vi "Edge Counting DAQ Assistant.vi"() -> ()   [LabVIEW 2020]
panel:
  out "Scalar":dbl
  in  "stop (F)":bool
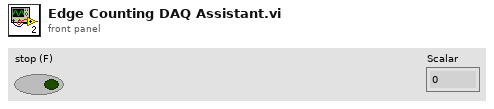
[diagram p1: front panel]
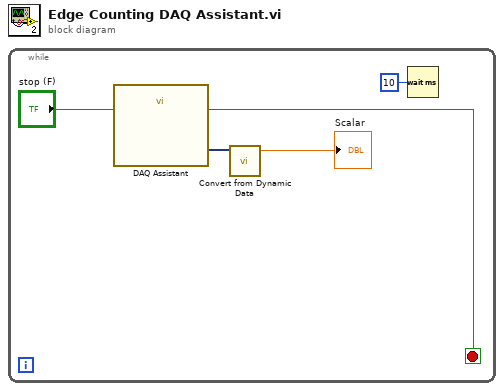
[diagram p0: block diagram]
diagram:
  n1 = while {
    stop <- w4 stop-if-true
    n2 = call "DAQ Assistant"("stop (F)"="stop (F)") -> ("data"=w3:dynamicdata, "stopped"=w4:bool)  [unwired: 15 in, 2 out]
    n3 = call "Convert from Dynamic Data"("Dynamic Data Type"=w3) -> ("Scalar"=→"Scalar":dbl)  [unwired: 3 in]
    n4 = Wait (ms)(milliseconds to wait=u32 10) -> ()  [unwired: 1 out]
  }
